vi "StatusSerialAdd.vi"(10 "Select":bool, 11 "Serial":u32) -> (3 "Serial":u32)   [LabVIEW 2020]
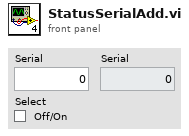
[diagram p1: front panel]
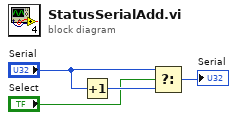
[diagram p0: block diagram]
diagram:
  n1 = Increment(x="Serial") -> (x+1=w4:u32)
  n2 = Select(t="Serial", s="Select", f=w4) -> (s? t:f=→"Serial":u32)
